vi "getStateName.vi"(9 "error in (no error)":errorcluster, 11 "initializable in":refnum<class "initializable.lvclass">) -> (1 "error out":errorcluster, 2 "State Name":string, 3 "initializable out":refnum<class "initializable.lvclass">)   [LabVIEW 2020, in "eos.lvlib" / "initializable.lvclass"]
uses:
  initializable.lvclass
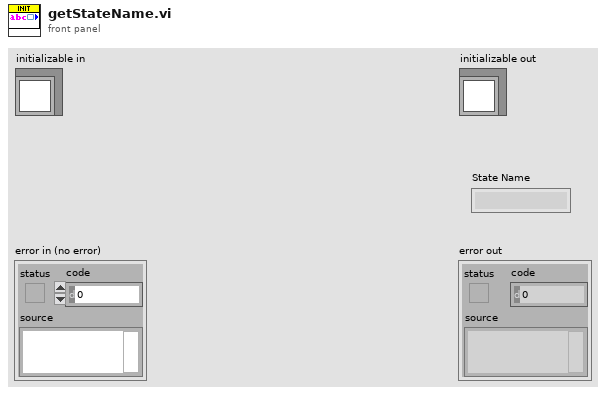
[diagram p1: front panel]
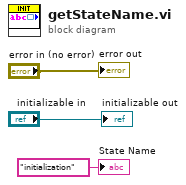
[diagram p0: block diagram]
diagram:
  "error out" <- "error in (no error)"
  "initializable out" <- "initializable in"
  "State Name" <- "initialization" ("State Name")
